vi "checkMAGStatus_eth.vi"(6 "mode (run)":enum16{"init", "run", "close"}(ring)=enum."run") -> (9 "DHSTB002":bool, 11 "BeamEnergy 2":dbl, 13 "DHSTB002 ok":bool, 14 "DHRTB101":bool, 15 "linacBeamEnergy":dbl, 16 "DHPTB101 ok":bool, 17 "DHSTB001":bool, 18 "BeamEnergy":dbl, 19 "DHSTB001 ok":bool)   [LabVIEW 2014]
panel:
  out "DHSTB002.status":i32
  out "DHSTB002.currentSetting":dbl
  out "DHSTB002.outputCurr":dbl
  out "DHSTB001.status":i32
  out "DHSTB001.currentSetting":dbl
  out "DHSTB001.outputCurr":dbl
  out "DHRTB101.outputCurr":dbl
  out "DHRTB101.currentSetting":dbl
  out "DHRTB101.status":i32
  out "error":bool=TRUE
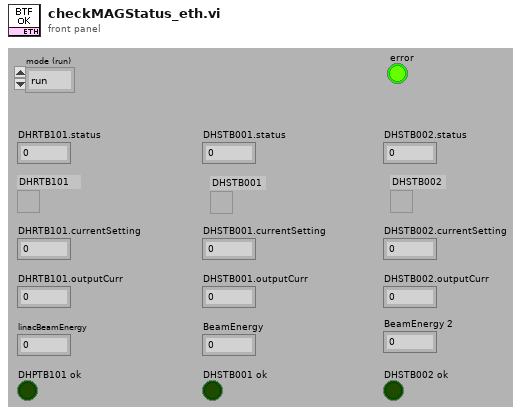
[diagram p1: front panel]
types:
  T1 = enum16{"init", "register [window]", "search [window]", "get [index]", "update [window, element]", "remove [window]"}
  T2 = typedef "UNIMagDyn.ctl" = cluster{"elemName":dbl, "consoleName":i32, "sysFlags":T3, "statusSetting":i32, "polaritySetting":i32, "currentSetting":dbl, "slewRateSetting":dbl, "cycleMode":i32, "statusReadout":i32, "polarityReadout":i32, "currentReadout":dbl, "slewRateReadout":dbl, "voltageReadout":dbl, "faults":u32[]}
  T3 = typedef "sysFlags.ctl" = cluster{"onLine":bool, "byPass":bool, "remote":bool, "busy":bool}
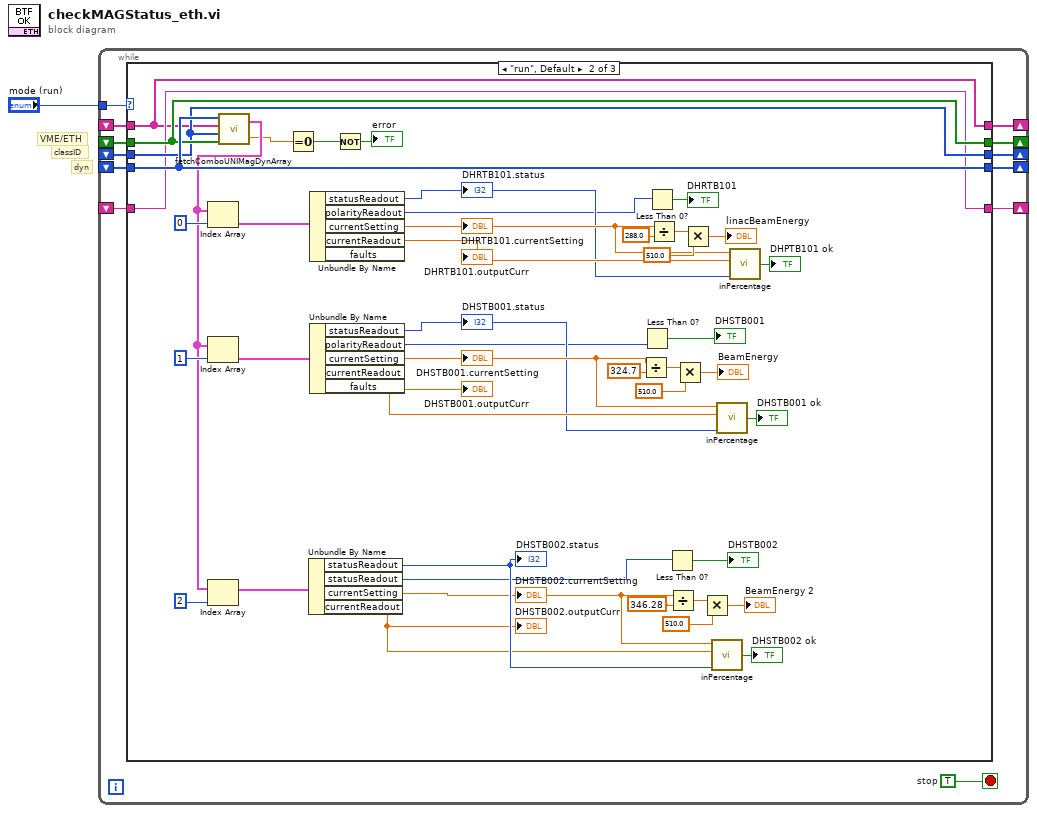
[diagram p0: block diagram]
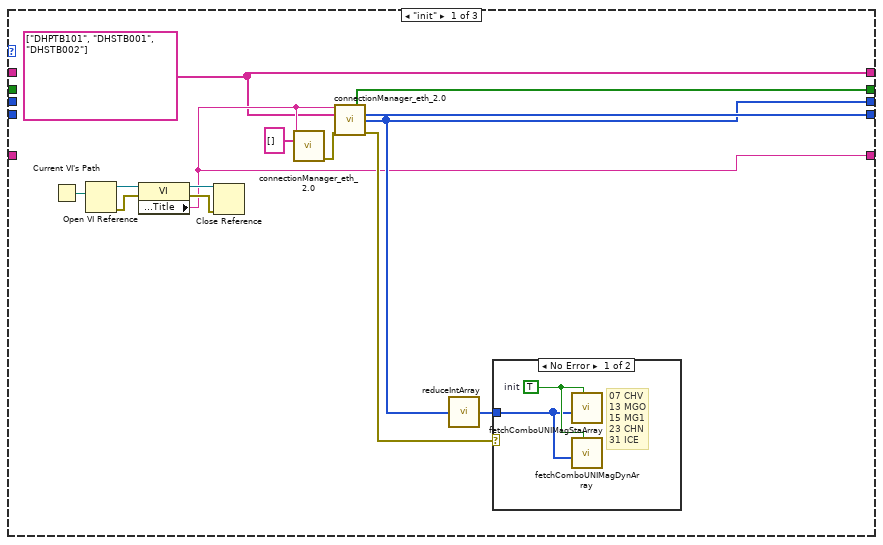
[diagram p2: hidden frame]
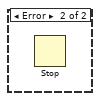
[diagram p3: hidden frame]
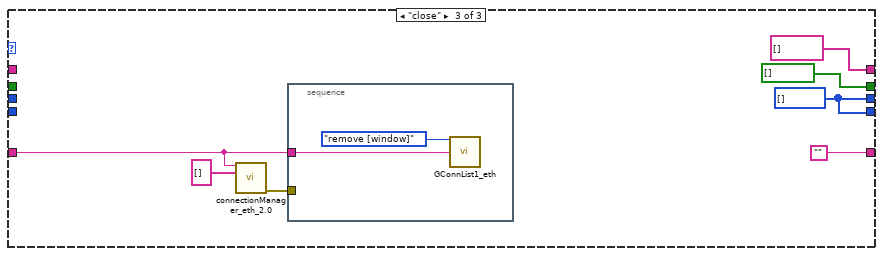
[diagram p4: hidden frame]
diagram:
  # "VME/ETH"
  # "classID"
  # "dyn"
  n1 = while {
    tunnel: "mode (run)" -> [w13]
    shift-right: [w12] -> _
    shift-left: _ -> [w11]
    shift-right: [w9] -> _
    shift-left: _ -> [w7]
    shift-right: [w8] -> _
    shift-left: _ -> [w6]
    shift-right: [w4] -> _
    shift-left: _ -> [w10]
    shift-right: [w3] -> _
    shift-left: _ -> [w2]
    stop <- w5 stop-if-true
    w5 = TRUE  # stop
    n2 = case shown="\"run\", Default" w13 {
      tunnel: [w24 w43 w79] -> w12
      tunnel: w11 -> [_ w43 _]
      tunnel: w10 -> [_ w31 w80]
      tunnel: [w25 w33 bool[] [] ("VME/ETH")] -> w9
      tunnel: [w22 w32 w79] -> w8
      tunnel: w7 -> [_ w33 _]
      tunnel: w6 -> [_ w32 _]
      tunnel: [w15 w31 ""] -> w4
      tunnel: [w14 w30 string[] []] -> w3
      tunnel: w2 -> [_ w30 _]
      frame "init" {
        w14 = string[] ["DHPTB101", "DHSTB001", "DHSTB002"]
        n3 = Current VI's Path() -> (path=w16:path)
        n4 = Open VI Reference(vi path=w16) -> (vi reference=w19:refnum<vi>, error out=w17:errorcluster)  [unwired: 5 in]
        n5 = property class="VI"(reference=w19, error in=w17) -> (reference out=w20:refnum<vi>, error out=w18:errorcluster, "Front Panel Window:Title"=w15:string)
        n6 = Close Reference(reference=w20, error in (no error)=w18) -> ()  [unwired: 1 out]
        n7 = call "connectionManager_eth_2.0.vi"("windowName"=w15, "elementList"=string[] []) -> ("errorOut"=w27:errorcluster)  [unwired: 9 in, 4 out]
        n8 = call "connectionManager_eth_2.0.vi"("windowName"=w15, "elementList"=w14, "errorIn"=w27) -> ("VME/ETH"=w25:bool[], "RTDBDynAdd"=w24:u32[], "classID"=w22:i32[], "errorOut"=w21:errorcluster)  [unwired: 8 in, 1 out]
        n9 = call "reduceIntArray.vi"("inputArray"=w22) -> ("reducedArray"=w23:i32[])
        n10 = case shown="No Error" w21 {
          tunnel: w23 -> [w28 _]
          frame No Error {
            w29 = TRUE  # init
            # "07 CHV\n13 MGO\n15 MG1\n23 CHN\n31 ICE"
            n11 = call "fetchComboUNIMagStaArray.vi"("classID"=w28, "init(F)"=w29) -> ()  [unwired: 3 in, 2 out]
            n12 = call "fetchComboUNIMagDynArray.vi"("classID"=w28, "init(F)"=w29) -> ()  [unwired: 3 in, 2 out]
          }
          frame Error {
            n13 = Stop() -> ()  [unwired: 1 in]
          }
        }
      }
      frame "run", Default {
        n14 = call "fetchComboUNIMagDynArray.vi"("RTDBDynAdd"=w43, "elementNameArray"=w30, "classID"=w32, "VME/ETH"=w33) -> ("uniformMagDynArray"=w37:T2[], "errorCode"=w35:cdb)  [unwired: 1 in]
        n15 = Index Array(array=w37, index=0 ("elemID")) -> (element=w41:T2)
        n16 = Index Array(array=w37, index=1 ("elemID")) -> (element=w39:T2)
        n17 = Index Array(array=w37, index=2 ("elemID")) -> (element=w36:T2)
        n18 = Equal To 0?(x=w35) -> (x = 0?=w34:bool)
        n19 = Unbundle By Name(w36) -> ("statusReadout"=w54:i32, "statusReadout"=w47:i32, "currentSetting"=w53:dbl, "currentReadout"=w52:dbl)
        "DHSTB002.status" <- w54
        "DHSTB002.currentSetting" <- w53
        "DHSTB002.outputCurr" <- w52
        n20 = Unbundle By Name(w41) -> ("statusReadout"=w60:i32, "polarityReadout"=w49:i32, "currentSetting"=w62:dbl, "currentReadout"=w61:dbl)  [unwired: 1 out]
        "DHRTB101.status" <- w60
        "DHRTB101.currentSetting" <- w62
        "DHRTB101.outputCurr" <- w61
        n21 = Unbundle By Name(w39) -> ("statusReadout"=w55:i32, "polarityReadout"=w48:i32, "currentSetting"=w57:dbl, "currentReadout"=w56:dbl)  [unwired: 1 out]
        "DHSTB001.status" <- w55
        "DHSTB001.currentSetting" <- w57
        "DHSTB001.outputCurr" <- w56
        n22 = Not(x=w34) -> (.not. x?=→"error":bool)
        n23 = Divide(x=w57, y=324.7) -> (x/y=w70:dbl)
        n24 = Less Than 0?(x=w48) -> (x < 0?=→"DHSTB001":bool)
        n25 = Less Than 0?(x=w49) -> (x < 0?=→"DHRTB101":bool)
        n26 = Divide(x=w62, y=288.0) -> (x/y=w73:dbl)
        n27 = Less Than 0?(x=w47) -> (x < 0?=→"DHSTB002":bool)
        n28 = Divide(x=w53, y=346.28) -> (x/y=w65:dbl)
        n29 = Multiply(x=w70, y=510.0) -> (x*y=→"BeamEnergy":dbl)
        n30 = Multiply(x=w73, y=510.0) -> (x*y=→"linacBeamEnergy":dbl)
        n31 = Multiply(x=w65, y=510.0) -> (x*y=→"BeamEnergy 2":dbl)
        n32 = call "inPercentage.vi"("set"=w53, "read"=w52, "stuatus"=w54) -> ("ok"=→"DHSTB002 ok":bool)  [unwired: 4 in]
        n33 = call "inPercentage.vi"("set"=w57, "read"=w56, "stuatus"=w55) -> ("ok"=→"DHSTB001 ok":bool)  [unwired: 4 in]
        n34 = call "inPercentage.vi"("set"=w62, "read"=w61, "stuatus"=w60) -> ("ok"=→"DHPTB101 ok":bool)  [unwired: 4 in]
      }
      frame "close" {
        w79 = i32[] [] ("classID")
        n35 = call "connectionManager_eth_2.0.vi"("windowName"=w80, "elementList"=string[] []) -> ("errorOut"=w76:errorcluster)  [unwired: 9 in, 4 out]
        n36 = stacked-sequence {
          tunnel: w80 -> [w82]
          tunnel: w76 -> [_]
          frame #0 {
            n37 = call "GConnList1_eth.vi"("mode (search)"=T1."remove [window]", "windowName"=w82) -> ()  [unwired: 10 in, 4 out]
          }
        }
      }
    }
  }
